vi "Names CRC.vi"(11 "Group in":refnum<class "Group.lvclass">) -> (2 "Names CRC":u32, 3 "Group out":refnum<class "Group.lvclass">)   [LabVIEW 2020, in "Vecto.lvlib" / "Group.lvclass"]
uses:
  Group.lvclass
  Group.lvclass/Group.ctl
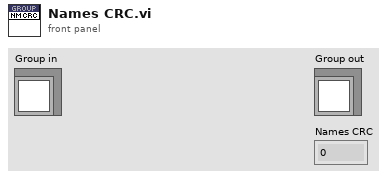
[diagram p1: front panel]
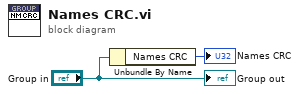
[diagram p0: block diagram]
diagram:
  n1 = Unbundle By Name("Group in") -> ("Names CRC"=→"Names CRC":u32)
  "Group out" <- "Group in"
